vi "test_OneSessOnePinGroupWithMorePinsOneInstrOneSiteReservation_CallNiDcPowerGetConnections1Pin1Connections_ReturnsError.vi"() -> (6 "pass":bool, 8 "result":string, 15 "error out":errorcluster)   [LabVIEW 2020, in "MeasurementServerTests.lvlib"]
uses:
  MeasurementServerTests.lvlib
  Runtime/MeasurementLink niDCPower/Get Connections - 1Pin 1Conn.vi
  Runtime/MeasurementLink niDCPower/MeasurementLink niDCPower.lvlib
panel:
  in  "error in":errorcluster
  # "Test assumes discovery service, pin map service, and session management service have already been started."
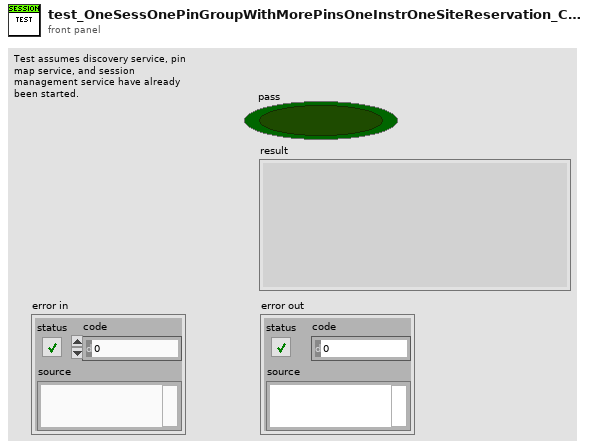
[diagram p1: front panel]
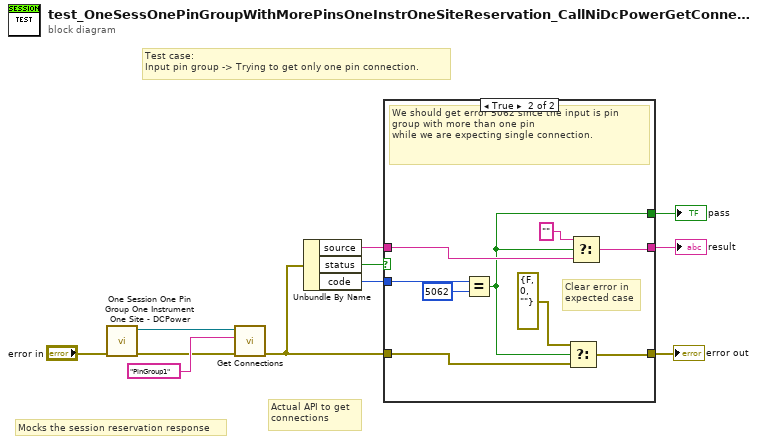
[diagram p0: block diagram]
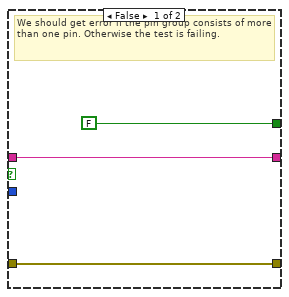
[diagram p2: hidden frame]
diagram:
  # "Actual API to get\nconnections"
  # "Mocks the session reservation response"
  # "Test case:\nInput pin group -> Trying to get only one pin connection."
  n1 = call "One Session One Pin Group One Instrument One Site - DCPower.vi"("error in"="error in") -> ("error out"=w8:errorcluster, "session reservation out"=w10:refnum<class "Session Reservation.lvclass">)  [unwired: 9 in]
  n2 = call-poly "Get Connections.vi"("error in"=w8, "pin or relay name"="PinGroup1", "session reservation in"=w10) -> ("error out"=w3:errorcluster)  [unwired: 6 in, 2 out]
  n3 = Unbundle By Name(w3) -> ("source"=w4:string, "status"=w5:bool, "code"=w2:i32)
  n4 = case shown="True" w5 {
    tunnel: [FALSE ("pass") w15] -> w7
    tunnel: [w12 w18] -> w6
    tunnel: w4 -> [w12 w16]
    tunnel: w3 -> [w13 w21]
    tunnel: w2 -> [_ w23]
    tunnel: [w13 w20] -> w1
    frame False {
      # "We should get error if the pin group consists of more than one pin. Otherwise the test is failing."
    }
    frame True {
      # "Clear error in\nexpected case"
      # "We should get error 5062 since the input is pin group with more than one pin\nwhile we are expecting single connection."
      n5 = Equal?(x=w23, y=5062) -> (x = y?=w15:bool)
      n6 = Select(t=errorcluster {"status"=FALSE, "code"=0, "source"=""}, s=w15, f=w21) -> (s? t:f=w20:errorcluster)
      n7 = Select(t="" ("source"), s=w15, f=w16) -> (s? t:f=w18:string)
    }
  }
  "error out" <- w1
  "pass" <- w7
  "result" <- w6
